vi "hwOperation_Get Devs Info.vi"(7 "hwType":string, 8 "error in":errorcluster, 9 "FirstSignalsOnly":bool=TRUE, 11 "hwDriverRef in":T1) -> (0 "error out":errorcluster, 2 "Devs Info":T2[](array[typedef]), 3 "hwDriverRef out":T1)   [LabVIEW 2016]
uses:
  DAQ-Config/Controls/PSCHN_Card Para.ctl
  DAQ-Config/Controls/PSCHN_Channel Para.ctl
  QX/hw_QX_hwDriverRef.ctl
  C:/Users/CL/Desktop/ZcDAQprj0811/ZcDAQprj/Modules/DAQ-Device/Hardware Drivers/QX/HBM LabVIEW Driver/DLLs/Hbm.Api.Common.dll
  QX/HBM LabVIEW Driver/DLLs/Hbm.Api.Common.dll
  Controls/hwSettings command.ctl
  C:/Users/CL/Desktop/ZcDAQprj0811/ZcDAQprj/Modules/DAQ-Device/Hardware Drivers/QX/HBM LabVIEW Driver/DLLs/Hbm.Api.LabVIEW.dll
  QX/HBM LabVIEW Driver/DLLs/Hbm.Api.LabVIEW.dll
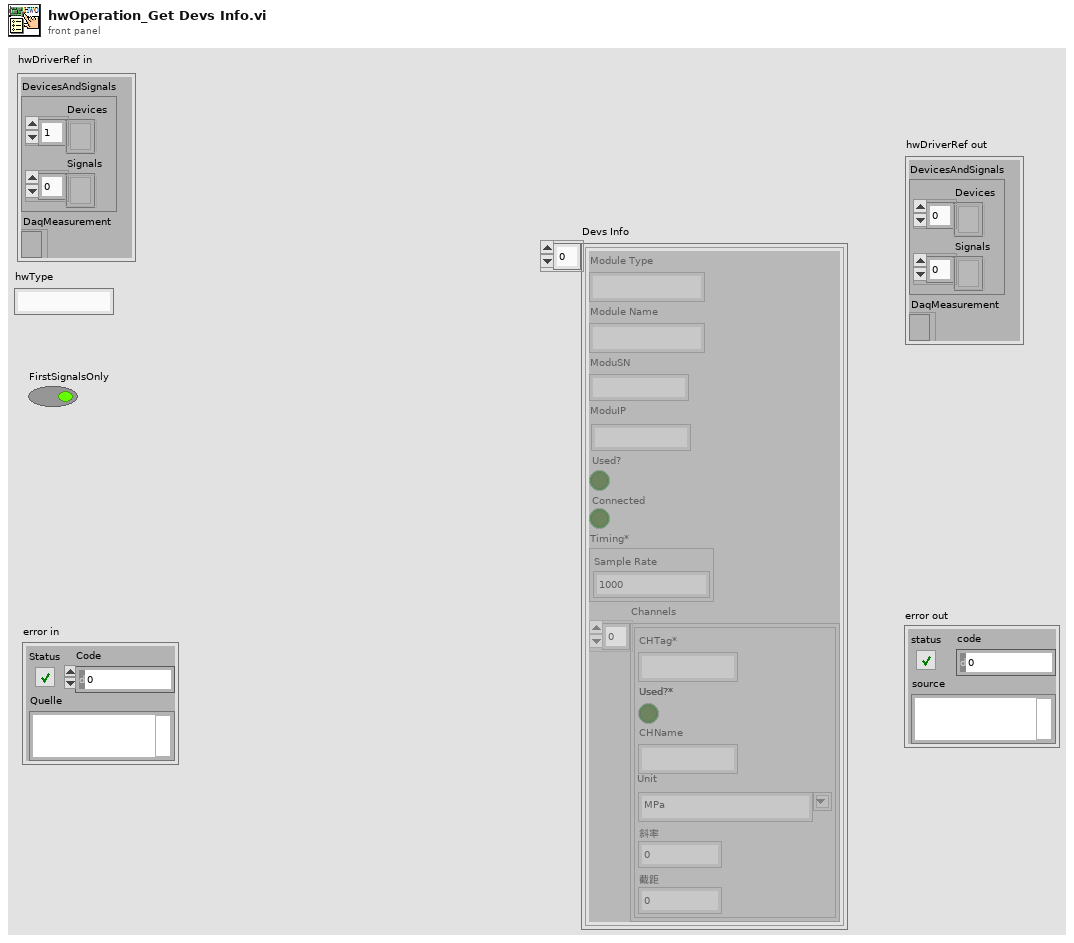
[diagram p1: front panel]
types:
  T1 = typedef "hw_QX_hwDriverRef.ctl" = cluster{"DevicesAndSignals":cluster{"Devices":refnum<k24>[], "Signals":refnum<k24>[]}, "DaqMeasurement":refnum<k24>}
  T2 = typedef "PSCHN_Card Para.ctl" = cluster{"Module Type":string, "Module Name":string, "ModuSN":string, "ModuIP":string, "Used?":bool, "Connected":bool, "Timing*":cluster{"Sample Rate":dbl}, "Channels":T3[]}
  T3 = typedef "PSCHN_Channel Para.ctl" = cluster{"CHTag*":string, "Used?*":bool, "CHName":string, "Unit":string, "斜率":dbl, "截距":dbl}
  T4 = typedef "hwSettings command.ctl" = enum16{"Init", "Read", "Clear"}
  T5 = typedef "hwDefaultSetting.ctl" = cluster{"hwType":string, "hwNumber":u32, "hwName":string[], "hwSN":string[], "hwCHNumber":u32[]}
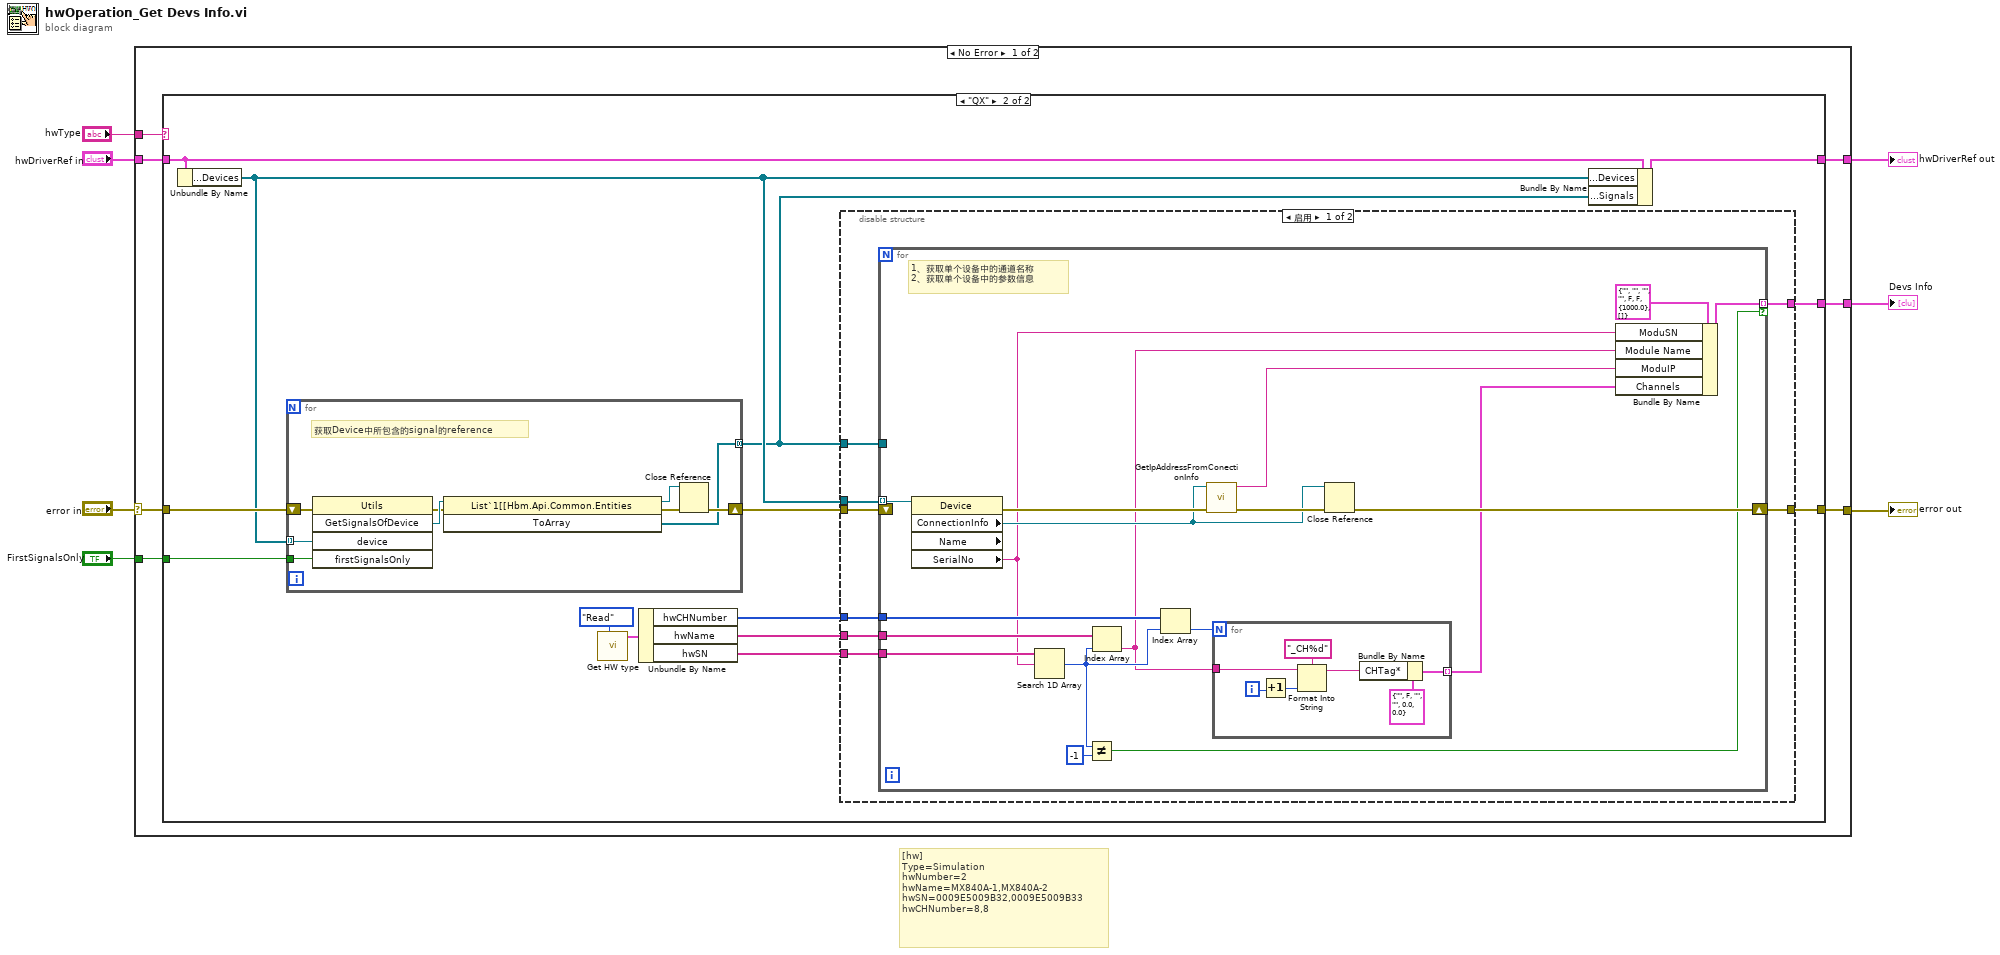
[diagram p0: block diagram]
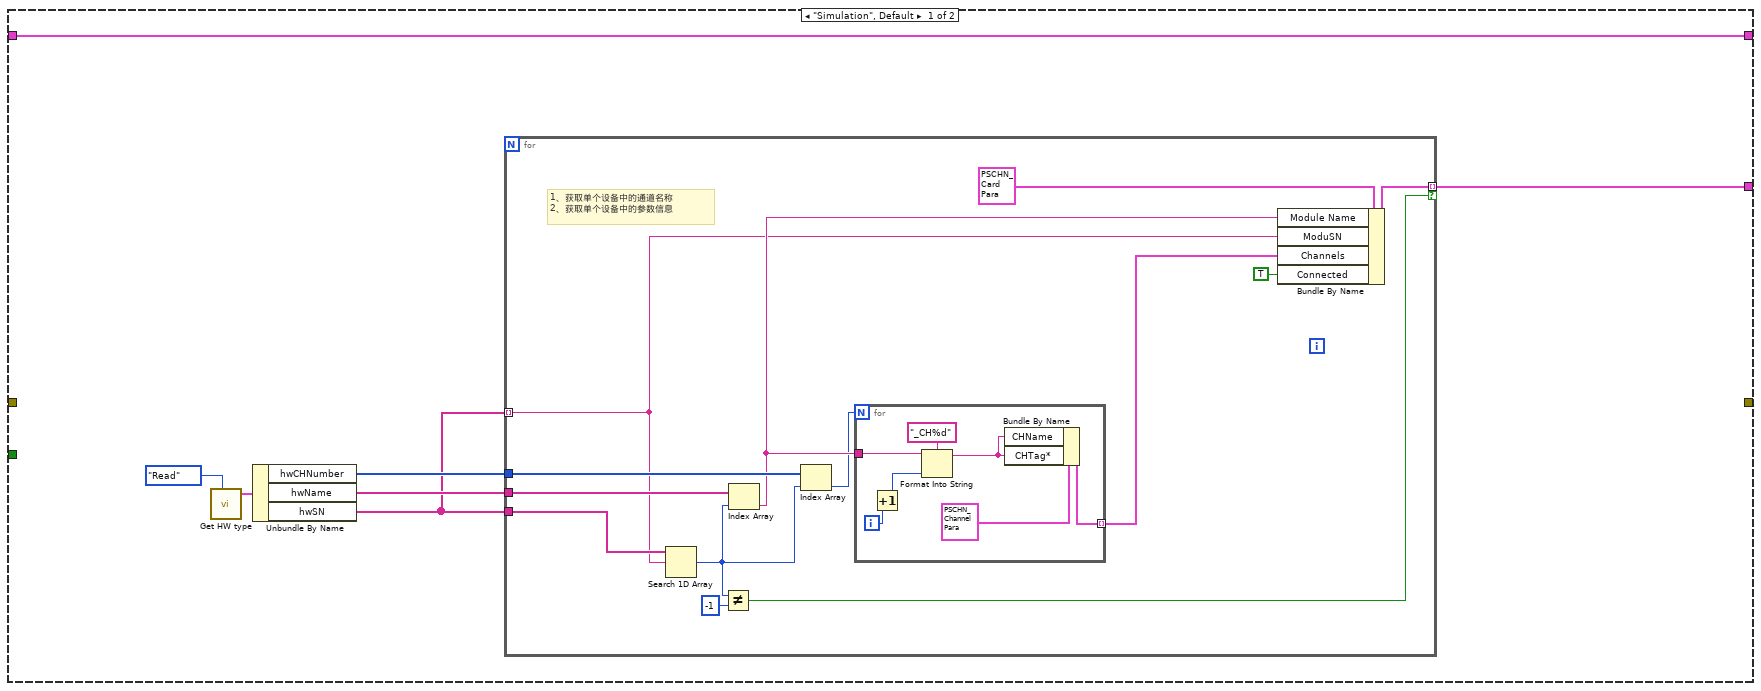
[diagram p2: hidden frame]
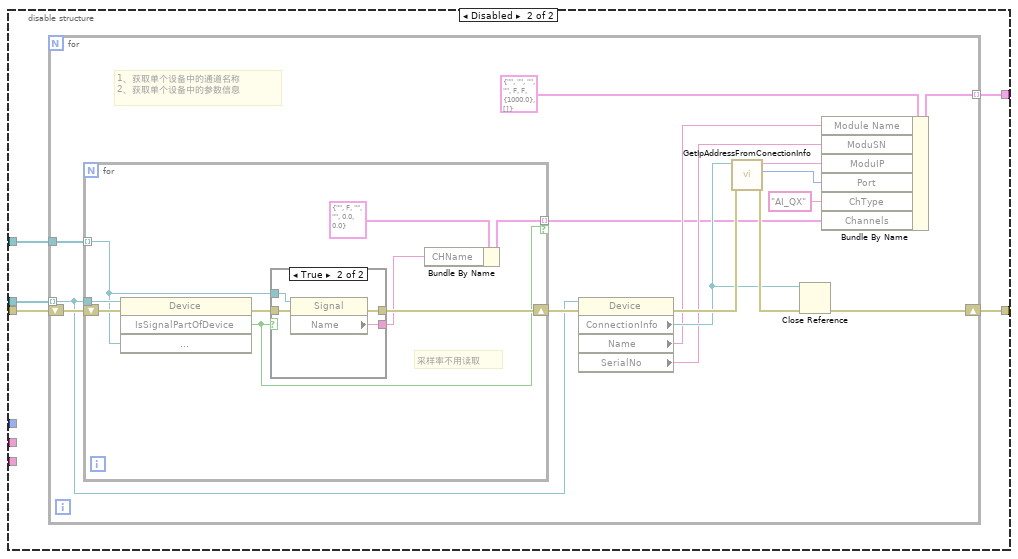
[diagram p3: hidden frame]
diagram:
  # "[hw]\nType=Simulation\nhwNumber=2\nhwName=MX840A-1,MX840A-2\nhwSN=0009E5009B32,0009E5009B33\nhwCHNumber=8,8"
  n1 = case shown="No Error" "error in" {
    selector: "error in" -> [w13 w134]
    tunnel: [w14 w134] -> w6
    tunnel: [w12 _] -> w4
    tunnel: "hwType" -> [w11 _]
    tunnel: "FirstSignalsOnly" -> [w10 _]
    tunnel: "hwDriverRef in" -> [w9 w133]
    tunnel: [w8 w133] -> w1
    frame No Error {
      n2 = case shown="\"QX\"" w11 {
        tunnel: [_ w52] -> w14
        tunnel: w13 -> [_ w51]
        tunnel: [w15 w55] -> w12
        tunnel: w10 -> [_ w54]
        tunnel: w9 -> [w21 w50]
        tunnel: [w21 w49] -> w8
        frame "Simulation", Default {
          n3 = call "Get HW type.vi"("Comm"=hwSettings_command."Read") -> ("hwDefaultSetting"=w19:T5)  [unwired: 9 in, 1 out]
          n4 = Unbundle By Name(w19) -> ("hwCHNumber"=w18:u32[], "hwName"=w17:string[], "hwSN"=w16:string[])
          n5 = for {
            tunnel: [w34] -> w15 mode=indexing if=w31
            tunnel: w16 -> [w33]
            tunnel: w17 -> [w29]
            tunnel: w18 -> [w30]
            tunnel: w16 -> [w24] mode=indexing
            # "1、获取单个设备中的通道名称\n2、获取单个设备中的参数信息"
            n6 = Search 1D Array(1D array=w33, element=w24) -> (index of element=w28:i32)  [unwired: 1 in]
            n7 = Not Equal?(x=w28, y=-1) -> (x != y?=w31:bool)
            n8 = Index Array(array=w29, index=w28) -> (element=w27:string)
            n9 = Index Array(array=w30, index=w28) -> (element=w26:u32)
            n10 = for {
              N: w26 -> [_]
              tunnel: w27 -> [w41]
              tunnel: [w37] -> w25 mode=indexing
              i -> [w40]
              n11 = Increment(x=w40) -> (x+1=w39:i32)
              n12 = Format Into String(format string="_CH%d", initial string=w41, w39) -> (resulting string=w35:string)  [unwired: 1 in, 1 out]
              n13 = Bundle By Name(cluster=T3 {"CHTag*"="MX840B-2_CH_1", "Used?*"=FALSE, "CHName"="", "Unit"="", "斜率"=0.0, "截距"=0.0} ("Channel"), "CHName"=w35, "CHTag*"=w35) -> (w37:T3)
            }
            n14 = Bundle By Name(cluster=T2 {"Module Type"="", "Module Name"="MX840B-2", "ModuSN"="0009E5009B32", "ModuIP"="158.168.8.11", "Used?"=FALSE, "Connected"=FALSE, "Timing*"={"Sample Rate"=1000.0}, "Channels"=[{"CHTag*"="MX840B-2_CH_1", "Used?*"=FALSE, "CHName"="", "Unit"="", "斜率"=0.0, "截距"=0.0}, {"CHTag*"="MX840B-2_CH_2", "Used?*"=FALSE, "CHName"="", "Unit"="", "斜率"=0.0, "截距"=0.0}, {"CHTag*"="MX840B-2_CH_3", "Used?*"=FALSE, "CHName"="", "Unit"="", "斜率"=0.0, "截距"=0.0}, {"CHTag*"="MX840B-2_CH_4", "Used?*"=FALSE, "CHName"="", "Unit"="", "斜率"=0.0, "截距"=0.0}, {"CHTag*"="MX840B-2_CH_5", "Used?*"=FALSE, "CHName"="", "Unit"="", "斜率"=0.0, "截距"=0.0}, {"CHTag*"="MX840B-2_CH_6", "Used?*"=FALSE, "CHName"="", "Unit"="", "斜率"=0.0, "截距"=0.0}, {"CHTag*"="MX840B-2_CH_7", "Used?*"=FALSE, "CHName"="", "Unit"="", "斜率"=0.0, "截距"=0.0}, {"CHTag*"="08", "Used?*"=FALSE, "CHName"="", "Unit"="", "斜率"=0.0, "截距"=0.0}]} ("Card"), "Module Name"=w27, "ModuSN"=w24, "Channels"=w25, "Connected"=TRUE) -> (w34:T2)
          }
        }
        frame "QX" {
          n15 = Unbundle By Name(w50) -> ("DevicesAndSignals.Devices"=w48:refnum<k24>[])
          n16 = for {
            shift-right: [w126] -> w53
            shift-left: w51 -> [w130]
            tunnel: w48 -> [w129] mode=indexing
            tunnel: w54 -> [w128]
            tunnel: [w124] -> w47 mode=concatenating
            # "获取Device中所包含的signal的reference"
            n17 = invoke on="Methodenknoten" class="Utils" method="GetSignalsOfDevice"(error in=w130, "device"=w129, "firstSignalsOnly"=w128) -> (error out=w131:errorcluster, "GetSignalsOfDevice"=w132:refnum<k24>)  [unwired: 2 in, 3 out]
            n18 = invoke on="Methodenknoten" class="List`1[[Hbm.Api.Common.Entities" method="ToArray"(reference=w132, error in=w131) -> (reference out=w125:refnum<k24>, error out=w127:errorcluster, "ToArray"=w124:refnum<k24>[])  [unwired: 1 in]
            n19 = Close Reference(reference=w125, error in (no error)=w127) -> (error out=w126:errorcluster)
          }
          n20 = call "Get HW type.vi"("Comm"=hwSettings_command."Read") -> ("hwDefaultSetting"=w45:T5)  [unwired: 9 in, 1 out]
          n21 = Unbundle By Name(w45) -> ("hwCHNumber"=w42:u32[], "hwName"=w43:string[], "hwSN"=w44:string[])
          n22 = disable-structure shown="启用" {
            disable-tunnel: [w63 w93] -> w55
            disable-tunnel: w53 -> [w62 w92]
            disable-tunnel: [w61 w91] -> w52
            disable-tunnel: w48 -> [w60 w90]
            disable-tunnel: w47 -> [w59 w89]
            disable-tunnel: w44 -> [w58 _]
            disable-tunnel: w43 -> [w57 _]
            disable-tunnel: w42 -> [w56 _]
            frame Enabled {
              n23 = for {
                tunnel: w60 -> [w76] mode=indexing
                shift-right: [w75] -> w61
                shift-left: w62 -> [_]
                tunnel: [w77] -> w63 mode=indexing if=w71
                tunnel: w59 -> [_]
                tunnel: w58 -> [w73]
                tunnel: w57 -> [w69]
                tunnel: w56 -> [w70]
                # "1、获取单个设备中的通道名称\n2、获取单个设备中的参数信息"
                n24 = property class="Device" props=["ConnectionInfo", "Name", "SerialNo"](reference=w76) -> (error out=w81:errorcluster, "ConnectionInfo"=w79:refnum<k24>, "SerialNo"=w64:string)  [unwired: 1 in, 2 out]
                n25 = Search 1D Array(1D array=w73, element=w64) -> (index of element=w68:i32)  [unwired: 1 in]
                n26 = Not Equal?(x=w68, y=-1) -> (x != y?=w71:bool)
                n27 = Index Array(array=w69, index=w68) -> (element=w65:string)
                n28 = Index Array(array=w70, index=w68) -> (element=w67:u32)
                n29 = call "GetIpAddressFromConectionInfo.vi"("Error in"=w81, "ConnectionInfo"=w79) -> ("Error out"=w80:errorcluster, "IpAddress"=w78:string)  [unwired: 7 in, 1 out]
                n30 = for {
                  N: w67 -> [_]
                  tunnel: w65 -> [w88]
                  tunnel: [w82] -> w66 mode=indexing
                  i -> [w87]
                  n31 = Increment(x=w87) -> (x+1=w86:i32)
                  n32 = Format Into String(format string="_CH%d", initial string=w88, w86) -> (resulting string=w84:string)  [unwired: 1 in, 1 out]
                  n33 = Bundle By Name(cluster=T3 {"CHTag*"="", "Used?*"=FALSE, "CHName"="", "Unit"="", "斜率"=0.0, "截距"=0.0} ("Channel"), "CHTag*"=w84) -> (w82:T3)
                }
                n34 = Close Reference(reference=w79, error in (no error)=w80) -> (error out=w75:errorcluster)
                n35 = Bundle By Name(cluster=T2 {"Module Type"="", "Module Name"="", "ModuSN"="", "ModuIP"="", "Used?"=FALSE, "Connected"=FALSE, "Timing*"={"Sample Rate"=1000.0}, "Channels"=[]} ("Card"), "ModuSN"=w64, "Module Name"=w65, "ModuIP"=w78, "Channels"=w66) -> (w77:T2)
              }
            }
            frame Disabled {
              n36 = for {
                tunnel: w90 -> [w98] mode=indexing
                shift-right: [w97] -> w91
                shift-left: w92 -> [w101]
                tunnel: [w104] -> w93 mode=indexing
                tunnel: w89 -> [w99]
                # "1、获取单个设备中的通道名称\n2、获取单个设备中的参数信息"
                n37 = for {
                  tunnel: w99 -> [w110] mode=indexing
                  shift-right: [w116] -> w100
                  shift-left: w101 -> [w118]
                  tunnel: w98 -> [w115]
                  tunnel: [w112] -> w95 mode=indexing if=w111
                  # "采样率不用读取"
                  n38 = invoke on="Methodenknoten" class="Device" method="IsSignalPartOfDevice"(reference=w115, error in=w118, "signalToCheck"=w110) -> (error out=w117:errorcluster, "IsSignalPartOfDevice"=w111:bool)  [unwired: 1 in, 2 out]
                  n39 = case shown="True" w111 {
                    tunnel: w117 -> [w119 w122]
                    tunnel: w110 -> [_ w123]
                    tunnel: [w119 w121] -> w116
                    tunnel: [_ w120] -> w113
                    frame False {
                    }
                    frame True {
                      n40 = property on="Eigenschaftsknoten" class="Signal"(reference=w123, error in=w122) -> (error out=w121:errorcluster, "Name"=w120:string)  [unwired: 1 out]
                    }
                  }
                  n41 = Bundle By Name(cluster=T3 {"CHTag*"="", "Used?*"=FALSE, "CHName"="", "Unit"="", "斜率"=0.0, "截距"=0.0} ("Channel"), "CHName"=w113) -> (w112:T3)
                }
                n42 = property class="Device"(reference=w98, error in=w100) -> (error out=w109:errorcluster, "ConnectionInfo"=w107:refnum<k24>, "Name"=w102:string, "SerialNo"=w105:string)  [unwired: 1 out]
                n43 = call "GetIpAddressFromConectionInfo.vi"("Error in"=w109, "ConnectionInfo"=w107) -> ("Error out"=w108:errorcluster, "Port"=w94:i32, "IpAddress"=w106:string)  [unwired: 7 in]
                n44 = Close Reference(reference=w107, error in (no error)=w108) -> (error out=w97:errorcluster)
                n45 = Bundle By Name(cluster=T2 {"Module Type"="", "Module Name"="", "ModuSN"="", "ModuIP"="", "Used?"=FALSE, "Connected"=FALSE, "Timing*"={"Sample Rate"=1000.0}, "Channels"=[]} ("Card"), "Module Name"=w102, "ModuSN"=w105, "ModuIP"=w106, "Port"=w94, "ChType"="AI_QX", "Channels"=w95) -> (w104:T2)
              }
            }
          }
          n46 = Bundle By Name(cluster=w50, "DevicesAndSignals.Devices"=w48, "DevicesAndSignals.Signals"=w47) -> (w49:T1)
        }
      }
    }
    frame Error {
    }
  }
  "error out" <- w6
  "Devs Info" <- w4
  "hwDriverRef out" <- w1
